vi "HVALS.vi"(8 "error in (no error)":errorcluster, 10 "key":string, 11 "Redis Client in":refnum<class "Redis Client.lvclass">) -> (0 "error out":errorcluster, 2 "RESP3 Value":variant, 3 "Redis Client out":refnum<class "Redis Client.lvclass">)   [LabVIEW 2023, in "Redis Client for LabVIEW.lvlib" / "Redis Client.lvclass"]
uses:
  Redis Client.lvclass
  lib/RESP3-for-LabVIEW/RESP3/subVIs/RESP3 Make String Base.vi
  lib/RESP3-for-LabVIEW/RESP3/types/RESP3 data type attribute.vi
  lib/RESP3-for-LabVIEW/RESP3/high-level/RESP3 Get Array.vi
  lib/RESP3-for-LabVIEW/RESP3/RESP3.lvlib
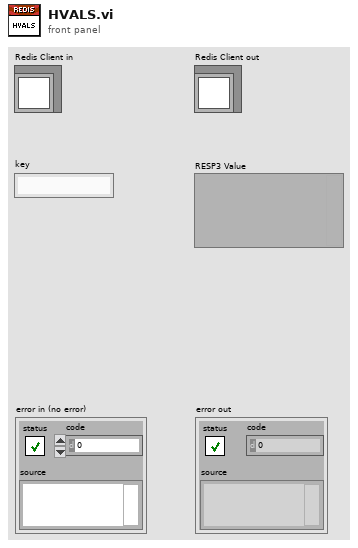
[diagram p1: front panel]
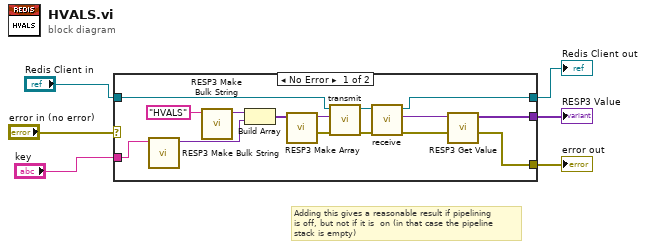
[diagram p0: block diagram]
diagram:
  # "Adding this gives a reasonable result if pipelining\nis off, but not if it is  on (in that case the pipeline\nstack is empty)"
  n1 = case shown="No Error" "error in (no error)" {
    selector: "error in (no error)" -> [_ w23]
    tunnel: [w7 w23] -> w5
    tunnel: "Redis Client in" -> [w21 w22]
    tunnel: [w14 w22] -> w3
    tunnel: "key" -> [w18 _]
    tunnel: [w9 _] -> w1
    frame No Error {
      n2 = call "RESP3 Make Bulk String.vi"("String"=w18) -> ("RESP3 Value out"=w17:variant)  [unwired: 9 in, 1 out]
      n3 = call "RESP3 Make Bulk String.vi"("String"="HVALS" ("string in")) -> ("RESP3 Value out"=w16:variant)  [unwired: 9 in, 1 out]
      n4 = Build Array(w16, w17) -> (w20:variant[])
      n5 = call "RESP3 Make Array.vi"("RESP3 Values in"=w20) -> ("error out"=w12:errorcluster, "RESP3 Value out"=w11:variant)  [unwired: 9 in]
      n6 = call-dynamic "transmit.vi"("error in (no error)"=w12, "RESP3 Value"=w11, "Redis Client in"=w21) -> ("error out"=w13:errorcluster, "Redis Client out"=w15:refnum<class "Redis Client.lvclass">)  [unwired: 7 in]
      n7 = call-dynamic "receive.vi"("error in (no error)"=w13, "Redis Client in"=w15) -> ("error out"=w8:errorcluster, "RESP3 Value"=w10:variant, "Redis Client out"=w14:refnum<class "Redis Client.lvclass">)  [unwired: 6 in, 1 out]
      n8 = call-poly "RESP3 Get Value.vi"("error in (no error)"=w8, "RESP3 Value in"=w10) -> ("error out"=w7:errorcluster, "RESP3 Values out"=w9:variant[])  [unwired: 6 in, 2 out]
    }
    frame Error {
    }
  }
  "error out" <- w5
  "Redis Client out" <- w3
  "RESP3 Value" <- w1
